vi "Simulator_WindTest.vi"() -> ()   [LabVIEW 2013]
doc: "This VI uses the wind simulator section of the simulator code for testing and demonstration purposes. Based on attraction conditions, the white noise generator output is pulled back to the set point linearly. (Basically a random walk with linear attraction back to set point). The set point can vary over time, it could be sinusoidal, linear, model of actual changing wind patterns, etc.\n\nMichael Bocamazo 2014/03/26"
panel:
  out "WindSpeed2":dbl
  out "Increment":dbl
  out "WindSpeed":dbl
  out "SetPoint":dbl
  out "AbsWind":dbl
  in  "stop":bool
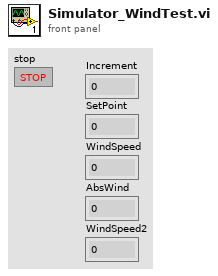
[diagram p1: front panel]
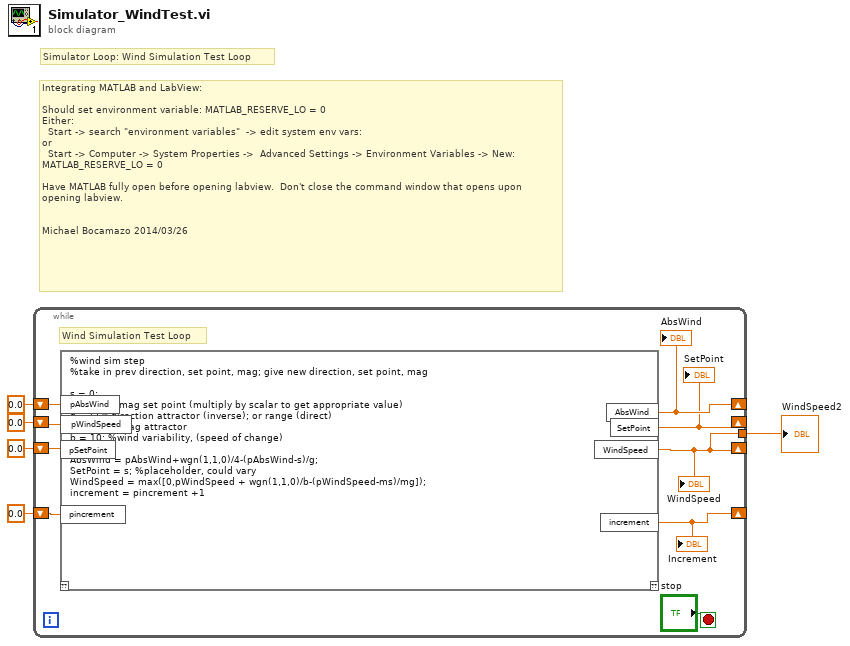
[diagram p0: block diagram]
diagram:
  # "Integrating MATLAB and LabView:\n\nShould set environment variable: MATLAB_RESERVE_LO = 0\nEither:\n  Start -> search \"environment variables\"  -> edit system env vars:\nor\n  Start -> Computer -> System Properties ->  Advanced Settings -> Environment Variables -> New:\nMATLAB_RESERVE_LO = 0 \n\nHave MATLAB fully open before opening labview.  Don't close the command window that opens upon opening labview.   \n\n\nMichael Bocamazo 2014/03/26"
  # "Simulator Loop: Wind Simulation Test Loop"
  n1 = while {
    shift-right: [w13] -> _
    shift-left: 0.0 -> [w14]
    shift-right: [w11] -> _
    shift-left: 0.0 -> [w12]
    shift-right: [w6] -> _
    shift-left: 0.0 -> [w10]
    shift-right: [w7] -> _
    shift-left: 0.0 -> [w8]
    tunnel: [w6] -> w1
    stop <- "stop" stop-if-true
    # "Wind Simulation Test Loop"
    n2 = script code="%wind sim step\n%take in prev direction, set point, mag; give new direction, set point, mag\n\ns = 0;\nms = 1; %mag set point (multiply by scalar to get appropriate value)\ng = 5; %direction attractor (inverse); or range (direct)\nmg = 5; %mag attractor\nb = 10; %wind variability, (speed of change)\n\nAbsWind = pAbsWind+wgn(1,1,0)/4-(pAbsWind-s)/g; \nSetPoint = s; %placeholder, could vary\nWindSpeed = max([0,pWindSpeed + wgn(1,1,0)/b-(pWindSpeed-ms)/mg]);\nincrement = pincrement +1"("pAbsWind"=w14, "pWindSpeed"=w12, "pSetPoint"=w10, "pincrement"=w8) -> ("AbsWind"=w13:dbl, "SetPoint"=w11:dbl, "WindSpeed"=w6:dbl, "increment"=w7:dbl)  [unwired: 1 in, 1 out]
    "AbsWind" <- w13
    "SetPoint" <- w11
    "WindSpeed" <- w6
    "Increment" <- w7
  }
  "WindSpeed2" <- w1
